vi "DSSwithFPO.vi"() -> ()   [LabVIEW 2023]
uses:
  Controls/Keys.ctl
  Controls/States.ctl
panel:
  out "LEDs":u32[](array[colorbox])
  out "Present state":T1
  in  "STOP":bool
  in  "Reset":bool
  in  "Keys":T2=[FALSE, FALSE, FALSE] caption="Keys inputs"
  # "K1    K2"
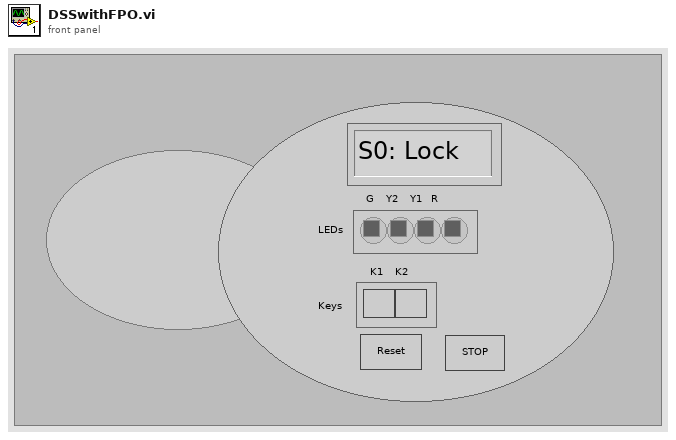
[diagram p1: front panel]
types:
  T1 = typedef "states.ctl" = enum16{"S0: Lock", "S1: Processing1 ", "S2: Processing2", "S3: Processing3", "S4: Unlock"}
  T2 = typedef "Keys.ctl" = bool[]
  T3 = typedef "States.ctl" = enum16{"S0: Lock", "S1: Processing1 ", "S2: Processing2", "S3: Processing3", "S4: Unlock"}
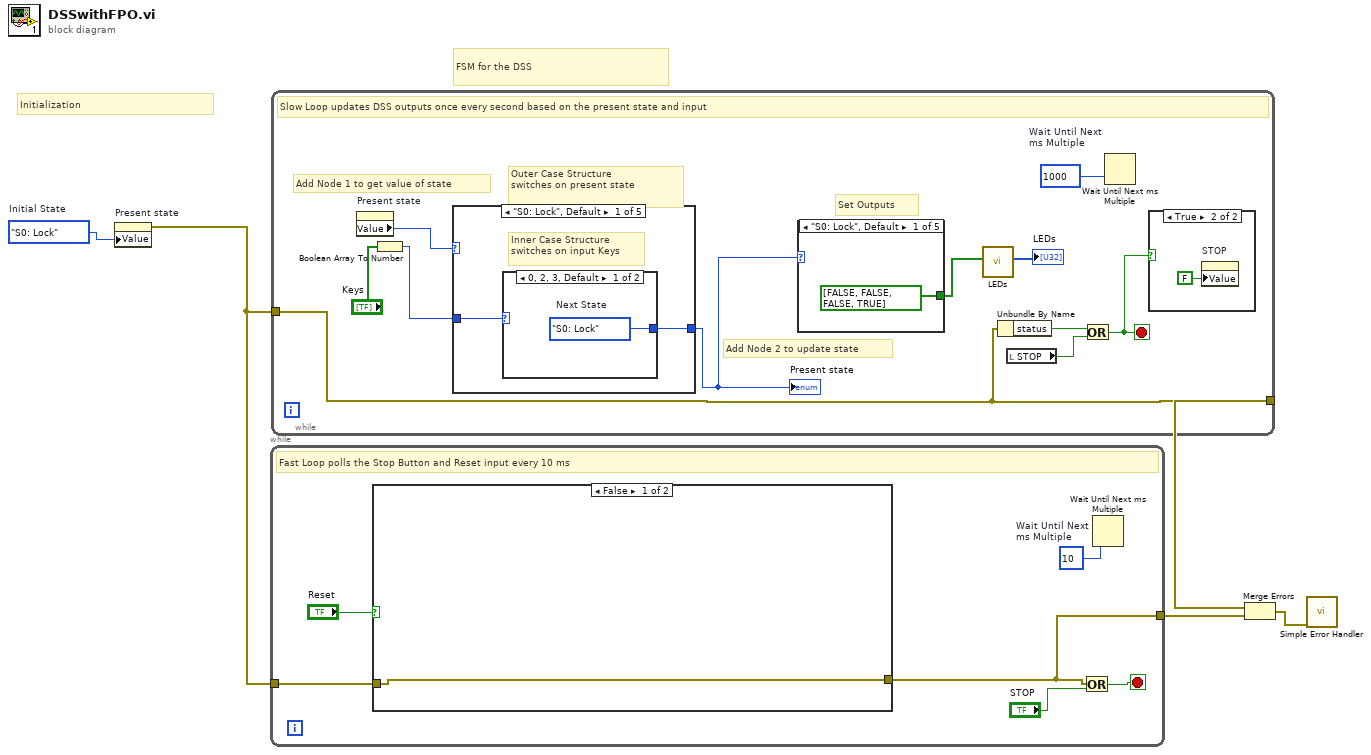
[diagram p0: block diagram]
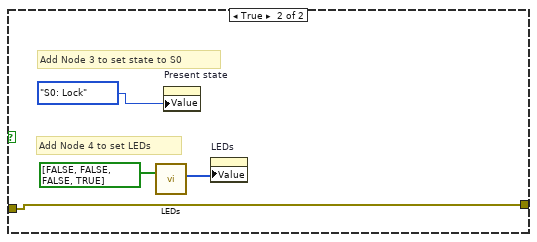
[diagram p2: hidden frame]
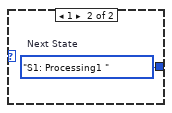
[diagram p4: hidden frame]
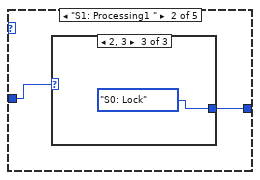
[diagram p5: hidden frame]
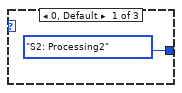
[diagram p6: hidden frame]
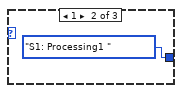
[diagram p7: hidden frame]
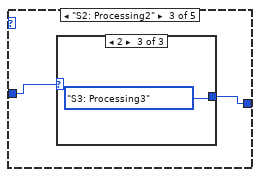
[diagram p8: hidden frame]
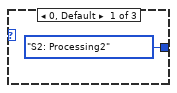
[diagram p9: hidden frame]
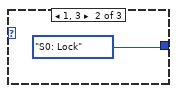
[diagram p10: hidden frame]
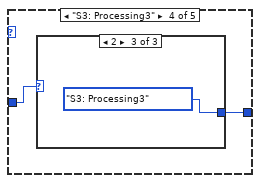
[diagram p11: hidden frame]
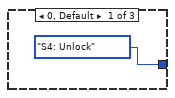
[diagram p12: hidden frame]
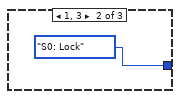
[diagram p13: hidden frame]
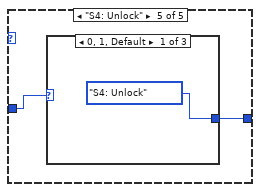
[diagram p14: hidden frame]
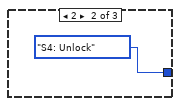
[diagram p15: hidden frame]
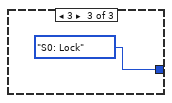
[diagram p16: hidden frame]
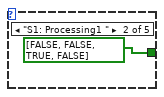
[diagram p17: hidden frame]
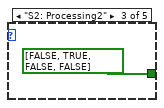
[diagram p18: hidden frame]
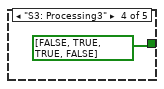
[diagram p19: hidden frame]
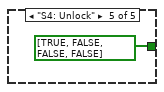
[diagram p20: hidden frame]
diagram:
  w4 = states."S0: Lock"  # Initial State
  # "Initialization"
  # "FSM for the DSS"
  n1 = property on="Present state" class="Enum (strict)"("Value"=w4) -> (error out=w5:errorcluster)  [unwired: 2 in, 1 out]
  n2 = while {
    tunnel: w5 -> [w9]
    tunnel: [w7] -> w3
    stop <- w11 stop-if-true
    # "Fast Loop polls the Stop Button and Reset input every 10 ms"
    n3 = case shown="False" "Reset" {
      tunnel: w9 -> [w12 w16]
      tunnel: [w12 w16] -> w7
      frame False {
      }
      frame True {
        # "Add Node 4 to set LEDs"
        # "Add Node 3 to set state to S0"
        n4 = call "LEDs.vi"("Array"=bool[] [FALSE, FALSE, FALSE, TRUE]) -> ("Array 2"=w14:u32[])  [unwired: 10 in]
        n5 = property on="Present state" class="Enum (strict)"("Value"=States."S0: Lock" ("State")) -> ()  [unwired: 2 in, 2 out]
        n6 = property on="LEDs" class="Arr (strict)"("Value"=w14) -> ()  [unwired: 2 in, 2 out]
      }
    }
    n7 = Or(x=w7, y="STOP") -> (x .or. y?=w11:bool)
    n8 = Wait Until Next ms Multiple "Wait Until Next \nms Multiple"(millisecond multiple=u32 10) -> ()  [unwired: 1 out]
  }
  n9 = while {
    tunnel: w5 -> [w18]
    tunnel: [w18] -> w2
    stop <- w17 stop-if-true
    # "Add Node 2 to update state"
    # "Add Node 1 to get value of state"
    # "Set Outputs"
    # "Outer Case Structure \nswitches on present state"
    # "Slow Loop updates DSS outputs once every second based on the present state and input"
    n10 = property on="Present state" class="Enum (strict)"() -> ("Value"=w19:T1)  [unwired: 2 in, 2 out]
    n11 = Boolean Array To Number(Boolean array="Keys") -> (number=w21:u32)
    n12 = case shown="\"S0: Lock\", Default" w19 {
      tunnel: [w30 w33 w38 w43 w48] -> w20
      tunnel: w21 -> [w29 w34 w39 w44 w49]
      frame "S0: Lock", Default {
        # "Inner Case Structure \nswitches on input Keys"
        n13 = case shown="0, 2, 3, Default" w29 {
          tunnel: [w31 w32] -> w30
          frame 0, 2, 3, Default {
            w31 = states."S0: Lock"  # Next State
          }
          frame 1 {
            w32 = states."S1: Processing1 "  # Next State
          }
        }
      }
      frame "S1: Processing1 " {
        n14 = case shown="2, 3" w34 {
          tunnel: [States."S2: Processing2" ("State") States."S1: Processing1 " ("State") States."S0: Lock" ("State")] -> w33
          frame 0, Default {
          }
          frame 1 {
          }
          frame 2, 3 {
          }
        }
      }
      frame "S2: Processing2" {
        n15 = case shown="2" w39 {
          tunnel: [States."S2: Processing2" ("State") States."S0: Lock" ("State") States."S3: Processing3" ("State")] -> w38
          frame 0, Default {
          }
          frame 1, 3 {
          }
          frame 2 {
          }
        }
      }
      frame "S3: Processing3" {
        n16 = case shown="2" w44 {
          tunnel: [States."S4: Unlock" ("State") States."S0: Lock" ("State") States."S3: Processing3" ("State")] -> w43
          frame 0, Default {
          }
          frame 1, 3 {
          }
          frame 2 {
          }
        }
      }
      frame "S4: Unlock" {
        n17 = case shown="0, 1, Default" w49 {
          tunnel: [States."S4: Unlock" ("State") States."S4: Unlock" ("State") States."S0: Lock" ("State")] -> w48
          frame 0, 1, Default {
          }
          frame 2 {
          }
          frame 3 {
          }
        }
      }
    }
    "Present state" <- w20
    n18 = case shown="\"S0: Lock\", Default" w20 {
      tunnel: [bool[] [FALSE, FALSE, FALSE, TRUE] bool[] [FALSE, FALSE, TRUE, FALSE] ("LEDs") bool[] [FALSE, TRUE, FALSE, FALSE] ("LEDs") bool[] [FALSE, TRUE, TRUE, FALSE] ("LEDs") bool[] [TRUE, FALSE, FALSE, FALSE] ("LEDs")] -> w25
      frame "S0: Lock", Default {
      }
      frame "S1: Processing1 " {
      }
      frame "S2: Processing2" {
      }
      frame "S3: Processing3" {
      }
      frame "S4: Unlock" {
      }
    }
    n19 = call "LEDs.vi"("Array"=w25) -> ("Array 2"=→"LEDs":u32[])  [unwired: 10 in]
    n20 = Unbundle By Name "Unbundle By Name"(w18) -> ("status"=w26:bool)
    n21 = local read "STOP"() -> (w27:bool)
    n22 = Or(x=w26, y=w27) -> (x .or. y?=w17:bool)
    n23 = Wait Until Next ms Multiple "Wait Until Next \nms Multiple"(millisecond multiple=u32 1000) -> ()  [unwired: 1 out]
    n24 = case shown="True" w17 {
      frame False {
      }
      frame True {
        n25 = property on="STOP" class="Bool (strict)"("Value"=FALSE ("STOP")) -> ()  [unwired: 2 in, 2 out]
      }
    }
  }
  n26 = Merge Errors(w2, w3) -> (w1:errorcluster)
  n27 = call <vilib>:"Simple Error Handler.vi"("error in (no error)"=w1) -> ()  [unwired: 4 in, 5 out]
